vi "Tracer_Level-Error.vi"(11 "Calltree Level":i32) -> (2 "Trace Enabled":bool, 3 "Category":string)   [LabVIEW 2018, in "TracerLibrary.lvlib" / "Tracer.lvclass"]
uses:
  Tracer.lvclass
  protected/Tracer_ClassAttributes.vi
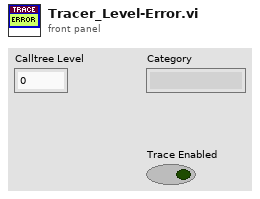
[diagram p1: front panel]
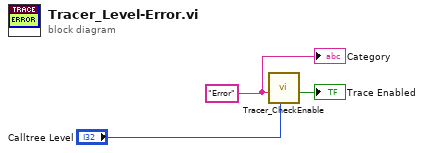
[diagram p0: block diagram]
diagram:
  w3 = "Error" ("Category")
  n1 = call "Tracer_CheckEnable.vi"("Calltree Level"="Calltree Level", "Category"=w3) -> ("Trace Enabled"=→"Trace Enabled":bool)  [unwired: 9 in]
  "Category" <- w3
